vi "ServoCommandPosition.vi"(0 "Device Reference":T1={"DeviceStatus"={"status"=FALSE, "code"=0, "source"=""}, "PWM Channel"=enum."Invalid", "DeadBand"={"Name"="", "maxPositivePwm"=0, "minPositivePwm"=0, "centerPwm"=0, "maxNegativePwm"=0, "minNegativePwm"=0, "angularRange"=0}}, 5 "Output Mode":T4(ring), 7 "Control Mode":enum16{"Safety", "Position"}(ring), 9 "Power or Testing Power":dbl, 11 "Error (in)":errorcluster) -> ()   [LabVIEW 2023]
doc: "Wrapper for commanding the power of a Talon FX motor controller. Supports voltage and safety interlock. Also supports the standard actuator testing interface and and the only sending new values on change."
uses:
  <vilib>/Rock Robotics/SystemInterfaces/DIO/FPGA_DIOPWMChannel.ctl
  <vilib>/Rock Robotics/WPI/PWM/WPI_PWMDeadband.ctl
  <vilib>/Rock Robotics/WPI/PWM/Servo/WPI_ServoDeviceRef.ctl
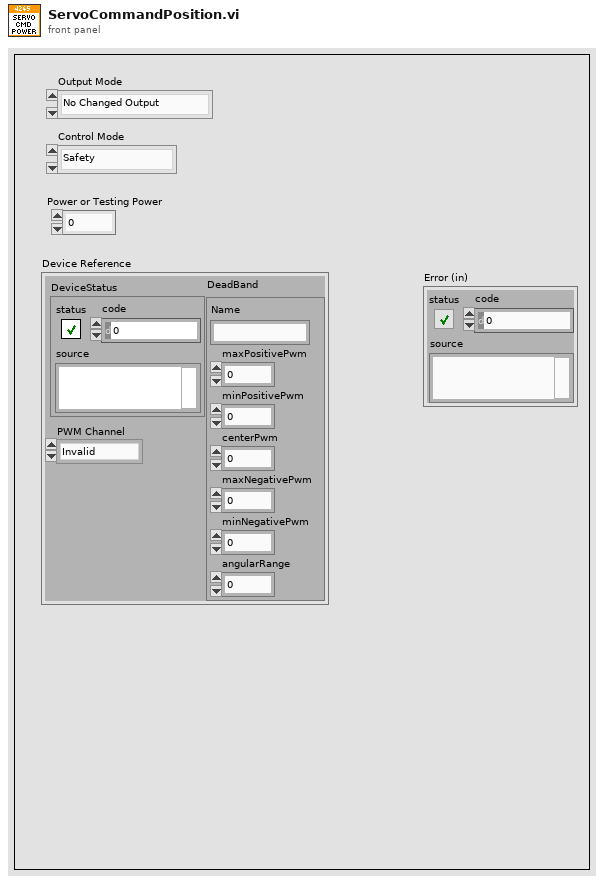
[diagram p1: front panel]
types:
  T1 = typedef "WPI_ServoDeviceRef.ctl" = cluster{"DeviceStatus":errorcluster, "PWM Channel":T2, "DeadBand":T3}
  T2 = typedef "FPGA_DIOPWMChannel.ctl" = enum8{"PWM 0", "PWM 1", "PWM 2", "PWM 3", "PWM 4", "PWM 5", "PWM 6", "PWM 7", "PWM 8", "PWM 9", "PWM MXP 0", "PWM MXP 1", "PWM MXP 2", "PWM MXP 3", "PWM MXP 4", "PWM MXP 5", "PWM MXP 6", "PWM MXP 7", "PWM MXP 8", "PWM MXP 9", "Invalid"}
  T3 = typedef "WPI_PWMDeadband.ctl" = cluster{"Name":string, "maxPositivePwm":i32, "minPositivePwm":i32, "centerPwm":i32, "maxNegativePwm":i32, "minNegativePwm":i32, "angularRange":u16}
  T4 = enum16{"No Changed Output", "New Normal Output", "New Testing Output"}
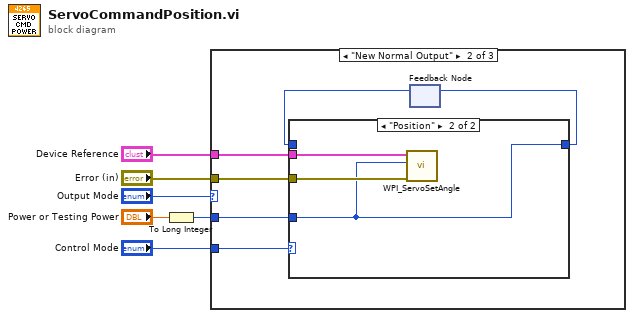
[diagram p0: block diagram]
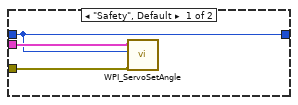
[diagram p3: hidden frame]
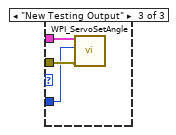
[diagram p4: hidden frame]
diagram:
  n1 = To Long Integer(number="Power or Testing Power") -> (32bit integer=w6:i32)
  n2 = case shown="\"New Normal Output\"" "Output Mode" {
    tunnel: w6 -> [_ w9 w20]
    tunnel: "Device Reference" -> [_ w12 w19]
    tunnel: "Control Mode" -> [_ w11 _]
    tunnel: "Error (in)" -> [_ w10 w21]
    frame "No Changed Output", Default {
    }
    frame "New Normal Output" {
      n3 = feedback #1() -> (w7:i32)  [unwired: 1 in]
      n4 = case shown="\"Position\"" w11 {
        tunnel: w12 -> [w15 w17]
        tunnel: w9 -> [_ w16]
        tunnel: w10 -> [w14 w18]
        tunnel: [w13 w16] -> w8
        tunnel: w7 -> [w13 _]
        frame "Safety", Default {
          n5 = call <vilib>:"WPI_ServoSetAngle.vi"("error in (no error)"=w14, "Angle"=w13, "ServoDeviceRef"=w15) -> ()  [unwired: 7 in, 2 out]
        }
        frame "Position" {
          n6 = call <vilib>:"WPI_ServoSetAngle.vi"("error in (no error)"=w18, "Angle"=w16, "ServoDeviceRef"=w17) -> ()  [unwired: 7 in, 2 out]
        }
      }
      n7 = feedback-in #1(w8) -> ()
    }
    frame "New Testing Output" {
      n8 = call <vilib>:"WPI_ServoSetAngle.vi"("error in (no error)"=w21, "Angle"=w20, "ServoDeviceRef"=w19) -> ()  [unwired: 7 in, 2 out]
    }
  }
